vi "Arrange VIWin - Resize FP.vi"(0 "VI in":refnum<vi>, 1 "FP objects arrangement info":T5, 2 "Window INI tokens":T4, 11 "error in":errorcluster) -> (15 "error out":errorcluster)   [LabVIEW 2017, in "Arrange VI Window.lvlib"]
uses:
  Arrange VI Window.lvlib
  <vilib>/Utility/miscctls.llb/LVRectTypeDef.ctl
  Arrange VIWin - FP Objects Arrangement Info.ctl
  Arrange VIWin - Window Gaps.ctl
  Arrange VIWin - Min Window Dimensions.ctl
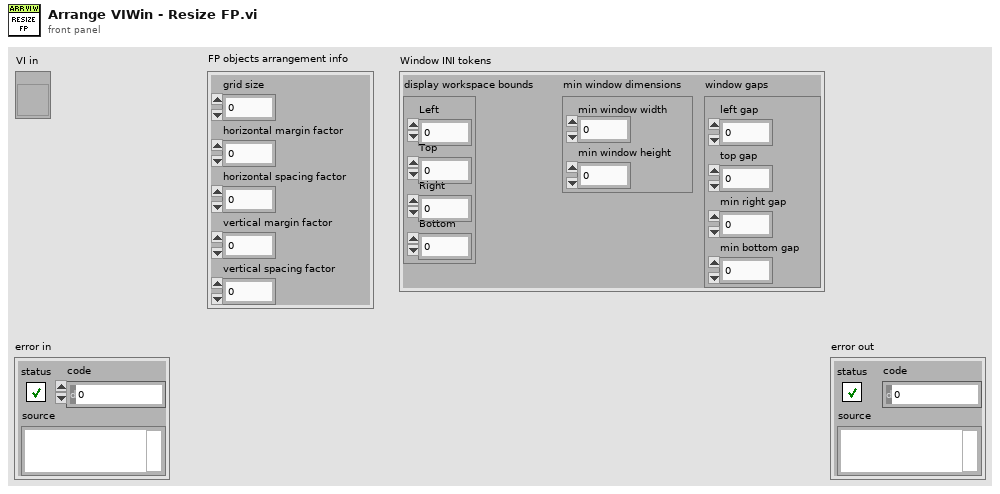
[diagram p1: front panel]
types:
  T1 = typedef "LVRectTypeDef.ctl" = cluster{"Left":i16, "Top":i16, "Right":i16, "Bottom":i16}
  T2 = typedef "Arrange VI Window.lvlib/Arrange VIWin - Min Window Dimensions.ctl" = cluster{"min window width":i16, "min window height":i16}
  T3 = typedef "Arrange VI Window.lvlib/Arrange VIWin - Window Gaps.ctl" = cluster{"left gap":i16, "top gap":i16, "min right gap":i16, "min bottom gap":i16}
  T4 = cluster{"display workspace bounds":T1, "min window dimensions":T2, "window gaps":T3}
  T5 = typedef "Arrange VI Window.lvlib/Arrange VIWin - FP Objects Arrangement Info.ctl" = cluster{"grid size":i32, "horizontal margin factor":i32, "horizontal spacing factor":i32, "vertical margin factor":i32, "vertical spacing factor":i32}
  T6 = enum32{"invalid VI type", "Standard VI", "Control VI", "Global VI", "Polymorphic VI", "Configuration VI", "SubSystem", "Facade VI", "Method VI", "Statechart Diagram VI"}
  T7 = typedef "LVPointTypeDef.ctl" = cluster{"Horizontal":i16, "Vertical":i16}
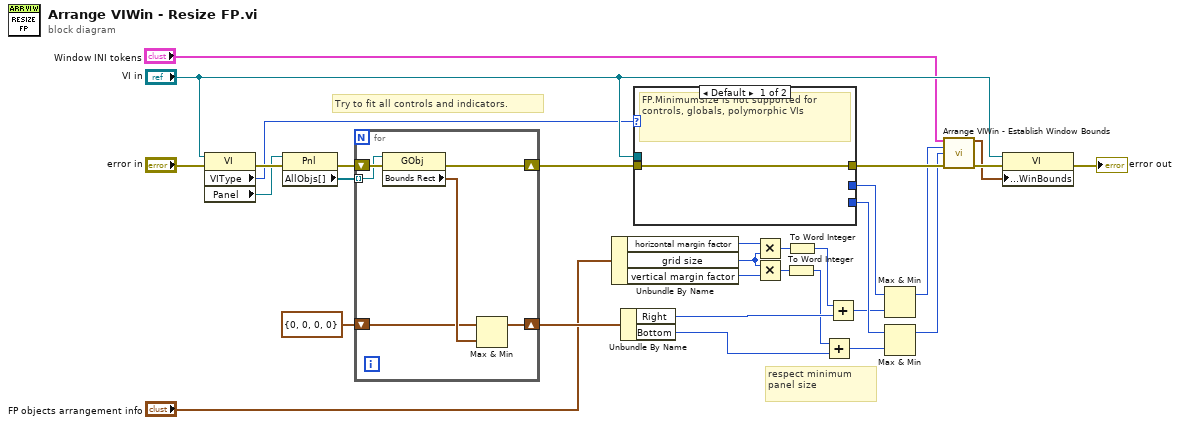
[diagram p0: block diagram]
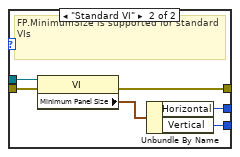
[diagram p2: hidden frame]
diagram:
  # "respect minimum panel size"
  # "Try to fit all controls and indicators."
  n1 = property class="VI"(reference="VI in", error in="error in") -> (error out=w29:errorcluster, "VIType"=w13:T6, "Panel"=w14:refnum<vi>)  [unwired: 1 out]
  n2 = property class="Pnl"(reference=w14, error in=w29) -> (error out=w26:errorcluster, "AllObjs[]"=w30:refnum<vi>[])  [unwired: 1 out]
  n3 = for {
    tunnel: w30 -> [w32] mode=indexing
    shift-right: [w36] -> w3
    shift-left: w26 -> [w37]
    shift-right: [w33] -> w24
    shift-left: T1 {"Left"=0, "Top"=0, "Right"=0, "Bottom"=0} ("Bounds Rect") -> [w34]
    n4 = property class="GObj"(reference=w32, error in=w37) -> (error out=w36:errorcluster, "Bounds Rect"=w35:T1)  [unwired: 1 out]
    n5 = Max & Min(x=w34, y=w35) -> (max(x,y)=w33:T1)  [unwired: 1 out]
  }
  n6 = Unbundle By Name("FP objects arrangement info") -> ("horizontal margin factor"=w12:i32, "grid size"=w9:i32, "vertical margin factor"=w8:i32)
  n7 = Unbundle By Name(w24) -> ("Right"=w23:i16, "Bottom"=w22:i16)
  n8 = case shown="Default" w13 {
    tunnel: [_ w44] -> w27
    tunnel: [_ w43] -> w25
    tunnel: "VI in" -> [_ w42]
    tunnel: w3 -> [w38 w41]
    tunnel: [w38 w40] -> w19
    frame Default {
      # "FP.MinimumSize is not supported for controls, globals, polymorphic VIs"
    }
    frame "Standard VI" {
      # "FP.MinimumSize is supported for standard VIs"
      n9 = property class="VI"(reference=w42, error in=w41) -> (error out=w40:errorcluster, "Minimum Panel Size"=w39:T7)  [unwired: 1 out]
      n10 = Unbundle By Name(w39) -> ("Horizontal"=w44:i16, "Vertical"=w43:i16)
    }
  }
  n11 = Multiply(x=w12, y=w9) -> (x*y=w10:i32)
  n12 = Multiply(x=w9, y=w8) -> (x*y=w7:i32)
  n13 = To Word Integer(number=w7) -> (16bit integer=w4:i16)
  n14 = To Word Integer(number=w10) -> (16bit integer=w5:i16)
  n15 = Add(x=w4, y=w22) -> (x+y=w11:i16)
  n16 = Add(x=w5, y=w23) -> (x+y=w6:i16)
  n17 = Max & Min(x=w27, y=w6) -> (max(x,y)=w17:i16)  [unwired: 1 out]
  n18 = Max & Min(x=w25, y=w11) -> (max(x,y)=w16:i16)  [unwired: 1 out]
  n19 = call "Arrange VIWin - Establish Window Bounds.vi"("Window INI tokens"="Window INI tokens", "content rectangle width"=w17, "content rectangle height"=w16, "error in"=w19) -> ("window bounds"=w15:T1, "error out"=w18:errorcluster)  [unwired: 10 in]
  n20 = property class="VI"(reference="VI in", error in=w18, "Front Panel.WinBounds"=w15) -> (error out=→"error out":errorcluster)  [unwired: 1 out]
